vi "Delete Install Files Missing From Source.vi"(8 "Error In":errorcluster, 11 "Configuration":T1) -> (0 "Error Out":errorcluster, 2 "Deleted From Souce":path[](array[path]), 3 "Configuration":T1)   [LabVIEW 2011, in "LVH-Build-Tools.lvlib"]
uses:
  LVH-Build-Tools.lvlib
  Type Defs/Configuration.ctl
  Type Defs/Install Configuration.ctl
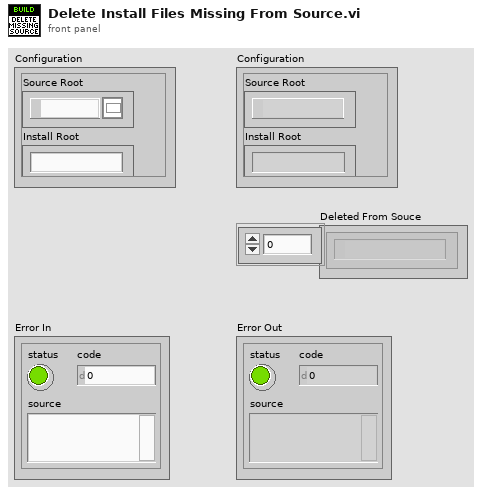
[diagram p1: front panel]
types:
  T1 = typedef "LVH-Build-Tools.lvlib/Configuration.ctl" = cluster{"Source Root":path, "Install Root":string, "Components":string[], "Ignore":string[], "Config Files":path[], "LV Directories":path[], "Install Paths":T2}
  T2 = typedef "LVH-Build-Tools.lvlib/Install Configuration.ctl" = cluster{"LabVIEW Directory":path, "Project Source Config":path}
  T3 = enum16{"Left Button", "Center Button", "Right Button", "Window Close"}
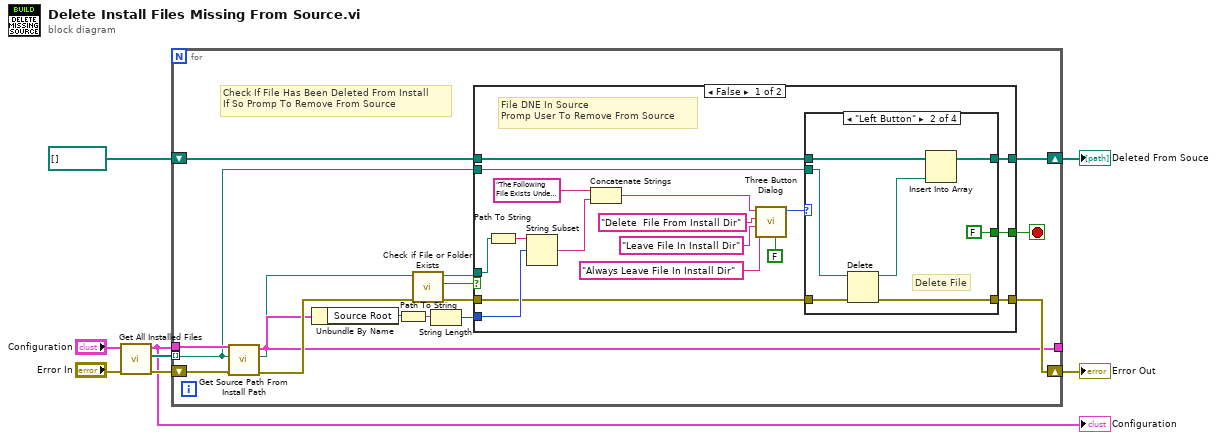
[diagram p0: block diagram]
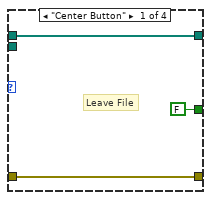
[diagram p2: hidden frame]
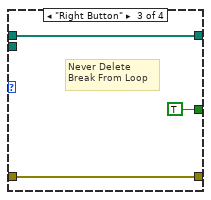
[diagram p3: hidden frame]
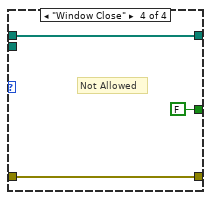
[diagram p4: hidden frame]
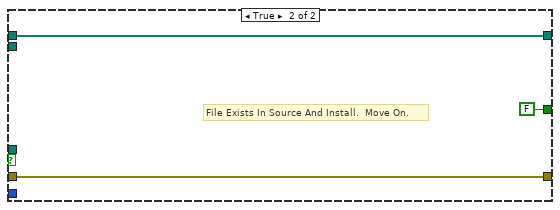
[diagram p5: hidden frame]
diagram:
  n1 = call "Get All Installed Files.vi"("Error In"="Error In", "Configuration"="Configuration") -> ("Error Out"=w4:errorcluster, "All Installed Files"=w5:path[], "Configuration"=w1:T1)  [unwired: 7 in]
  "Configuration" <- w1
  n2 = for {
    tunnel: w5 -> [w12] mode=indexing
    shift-right: [w21] -> w8
    shift-left: w4 -> [w18]
    tunnel: [w16] -> _
    shift-right: [w19] -> w7
    shift-left: path[] [] ("Array in") -> [w20]
    tunnel: w1 -> [w13]
    stop <- w11 stop-if-true
    # "Check If File Has Been Deleted From Install \nIf So Promp To Remove From Source"
    n3 = call "Get Source Path From Install Path.vi"("Error In"=w18, "Install File Path"=w12, "Configuration"=w13) -> ("Error Out"=w17:errorcluster, "Install File Path"=w14:path, "Configuraiton"=w16:T1)  [unwired: 5 in, 1 out]
    n4 = Unbundle By Name(w16) -> ("Source Root"=w10:path)
    n5 = Path To String(path=w10) -> (string=w9:string)
    n6 = call <vilib>:"Check if File or Folder Exists.vi"("error in (no error)"=w17, "path"=w14) -> ("error out"=w23:errorcluster, "file or folder exists?"=w24:bool, "dup path"=w15:path)  [unwired: 7 in]
    n7 = String Length(string=w9) -> (length=w22:i32)
    n8 = case shown="False" w24 {
      tunnel: w23 -> [w37 w60]
      tunnel: w22 -> [w41 _]
      tunnel: [w36 w60] -> w21
      tunnel: w20 -> [w35 w59]
      tunnel: [w34 w59] -> w19
      tunnel: w12 -> [w32 _]
      tunnel: w15 -> [w31 _]
      tunnel: [w25 FALSE] -> w11
      frame False {
        # "File DNE In Source\nPromp User To Remove From Source"
        n9 = Path To String(path=w31) -> (string=w33:string)
        n10 = String Subset(string=w33, offset (0)=w41) -> (substring=w40:string)  [unwired: 1 in]
        n11 = Concatenate Strings("The Following File Exists Under The Install Directory But Not The Source Directory.  If you choose not to delete this file it will be synced with the source directory next time you run Sync Source.vi\n\n", w40) -> (w39:string)
        n12 = call <vilib>:"Three Button Dialog.vi"("Allow user to close window? (TRUE)"=FALSE, "Right Button Text (\"Cancel\")"="Always Leave File In Install Dir" ("F button name (\"Cancel\")"), "Center Button Text (\"No\")"="Leave File In Install Dir" ("F button name (\"Cancel\")"), "Left Button Text (\"Yes\")"="Delete  File From Install Dir" ("T button name (\"OK\")"), "message"=w39) -> ("Which Button?"=w38:T3)  [unwired: 6 in]
        n13 = case shown="\"Left Button\"" w38 {
          tunnel: w37 -> [w44 w51 w52 w55]
          tunnel: [w44 w50 w52 w55] -> w36
          tunnel: w35 -> [w43 w49 w53 w57]
          tunnel: [w43 w47 w53 w57] -> w34
          tunnel: w32 -> [_ w46 _ _]
          tunnel: [FALSE FALSE TRUE FALSE] -> w25
          frame "Center Button" {
            # "Leave File"
          }
          frame "Left Button" {
            # "Delete File"
            n14 = Delete(path (use dialog)=w46, error in=w51) -> (deleted path=w48:path, error out=w50:errorcluster)  [unwired: 3 in, 1 out]
            n15 = Insert Into Array(array=w49, new element=w48) -> (w47:path[])  [unwired: 1 in]
          }
          frame "Right Button" {
            # "Never Delete\nBreak From Loop"
          }
          frame "Window Close" {
            # "Not Allowed"
          }
        }
      }
      frame True {
        # "File Exists In Source And Install.  Move On."
      }
    }
  }
  "Error Out" <- w8
  "Deleted From Souce" <- w7
